vi "GUARDADO_SQL.vi"(4 "date string":string, 5 "time string":string, 6 "BOMBA":string, 7 "PORCENTAJE_TANQUE":dbl, 9 "ALARMA":string, 10 "ESTADO TANQUE":string, 11 "VELOCIDAD_LLENADO":dbl) -> ()   [LabVIEW 2019, in "GUARDAR_DATOS_SQL.lvlib"]
uses:
  GUARDAR_DATOS_SQL/GUARDAR_DATOS_SQL.lvlib
  <vilib>/drjdpowell/SQLite Library/SQL Connection/Open (path).vi
  <vilib>/drjdpowell/SQLite Library/SQL Connection/Open (string).vi
  <vilib>/AdvancedString/Path To Command Line String.vi
  <vilib>/drjdpowell/SQLite Library/SQL Connection/Execute SQL (No results).vi
  <vilib>/drjdpowell/SQLite Library/SQL Connection/Connection.lvclass
  <vilib>/drjdpowell/SQLite Library/SQLite.lvlib
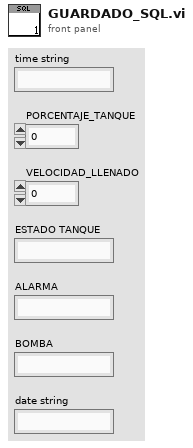
[diagram p1: front panel]
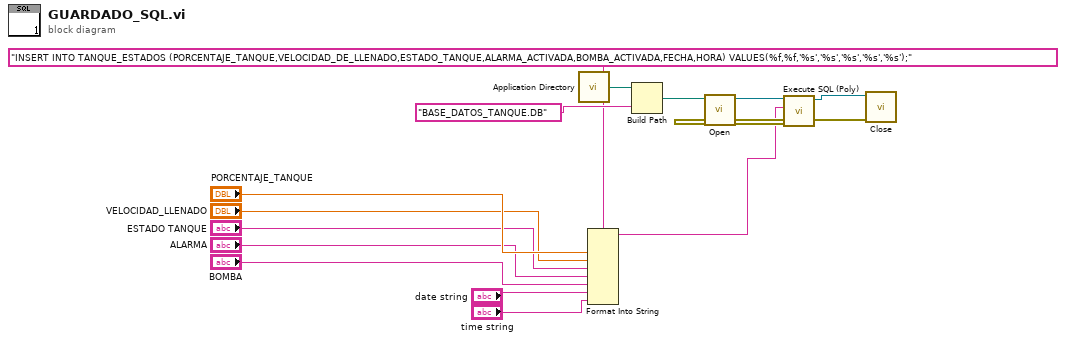
[diagram p0: block diagram]
diagram:
  n1 = call <vilib>:"Application Directory.vi"() -> ("Application Directory"=w10:path)
  n2 = Format Into String(format string="INSERT INTO TANQUE_ESTADOS (PORCENTAJE_TANQUE,VELOCIDAD_DE_LLENADO,ESTADO_TANQUE,ALARMA_ACTIVADA,BOMBA_ACTIVADA,FECHA,HORA) VALUES(%f,%f,'%s','%s','%s','%s','%s');", "PORCENTAJE_TANQUE", "VELOCIDAD_LLENADO", "ESTADO TANQUE", "ALARMA", "BOMBA", "date string", "time string") -> (resulting string=w6:string)  [unwired: 2 in, 1 out]
  n3 = Build Path(base path=w10, name or relative path="BASE_DATOS_TANQUE.DB") -> (appended path=w12:path)
  n4 = call-poly <vilib>:"Open.vi"("db file"=w12) -> ("error out"=w15:errorcluster, "SQLite Connection"=w13:refnum<class "Connection.lvclass">)  [unwired: 9 in]
  n5 = call-poly <vilib>:"Execute SQL (Poly).vi"("error in (no error)"=w15, "SQL"=w6, "SQLite Connection in"=w13) -> ("error out"=w16:errorcluster, "SQLite Connection"=w14:refnum<class "Connection.lvclass">)  [unwired: 7 in]
  n6 = call-dynamic "Close.vi"("error in (no error)"=w16, "SQLite Connection in"=w14) -> ()  [unwired: 9 in, 1 out]
